vi "SSH_writeRead.vi"(4 "Timeout":u32=5000, 6 "EOL":string="$", 7 "Text":string, 8 "error in (no error)":errorcluster, 10 "Console In":string, 11 "Python in":cluster{"Python":refnum<k35>, "py file":path}) -> (0 "error out":errorcluster, 2 "Console Out":string, 3 "Python out":cluster{"Python":refnum<k35>, "py file":path})   [LabVIEW 2020]
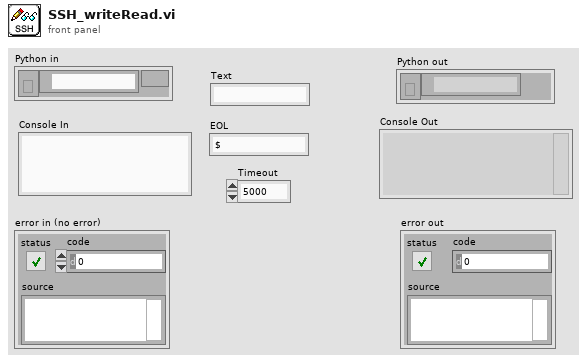
[diagram p1: front panel]
types:
  T1 = cluster{"session out":refnum<k35>, "py file":path}
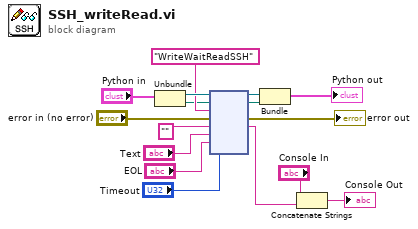
[diagram p0: block diagram]
diagram:
  n1 = Unbundle("Python in") -> ("Python"=w11:refnum<k35>, "py file"=w2:path)
  n2 = node(w11, w2, "WriteWaitReadSSH" ("function name"), "error in (no error)", "" ("function name"), "Text", "EOL", "Timeout") -> (w5:refnum<k35>, →"error out":errorcluster, w8:string)  [unwired: 3 in, 2 out]
  n3 = Bundle("session out"=w5, "py file"=w2) -> (→"Python out":T1)  [unwired: 1 in]
  n4 = Concatenate Strings("Console In", w8) -> (→"Console Out":string)
